vi "Untitled 1.vi"() -> ()   [LabVIEW 2017]
uses:
  <vilib>/xml/Load XML String.vi
  <vilib>/xml/Close Reference(Node).vi
  <vilib>/addons/internet/NI_InternetTK_Core_VIs.lvlib
  <vilib>/xml/NI_XML.lvlib
  <resource>/objmgr/DOMUserDefRef.rc
panel:
  out "I, J,K,X, Y,Z":dbl[](array[numeric])
  out "content":string
  out "concatenated string":string
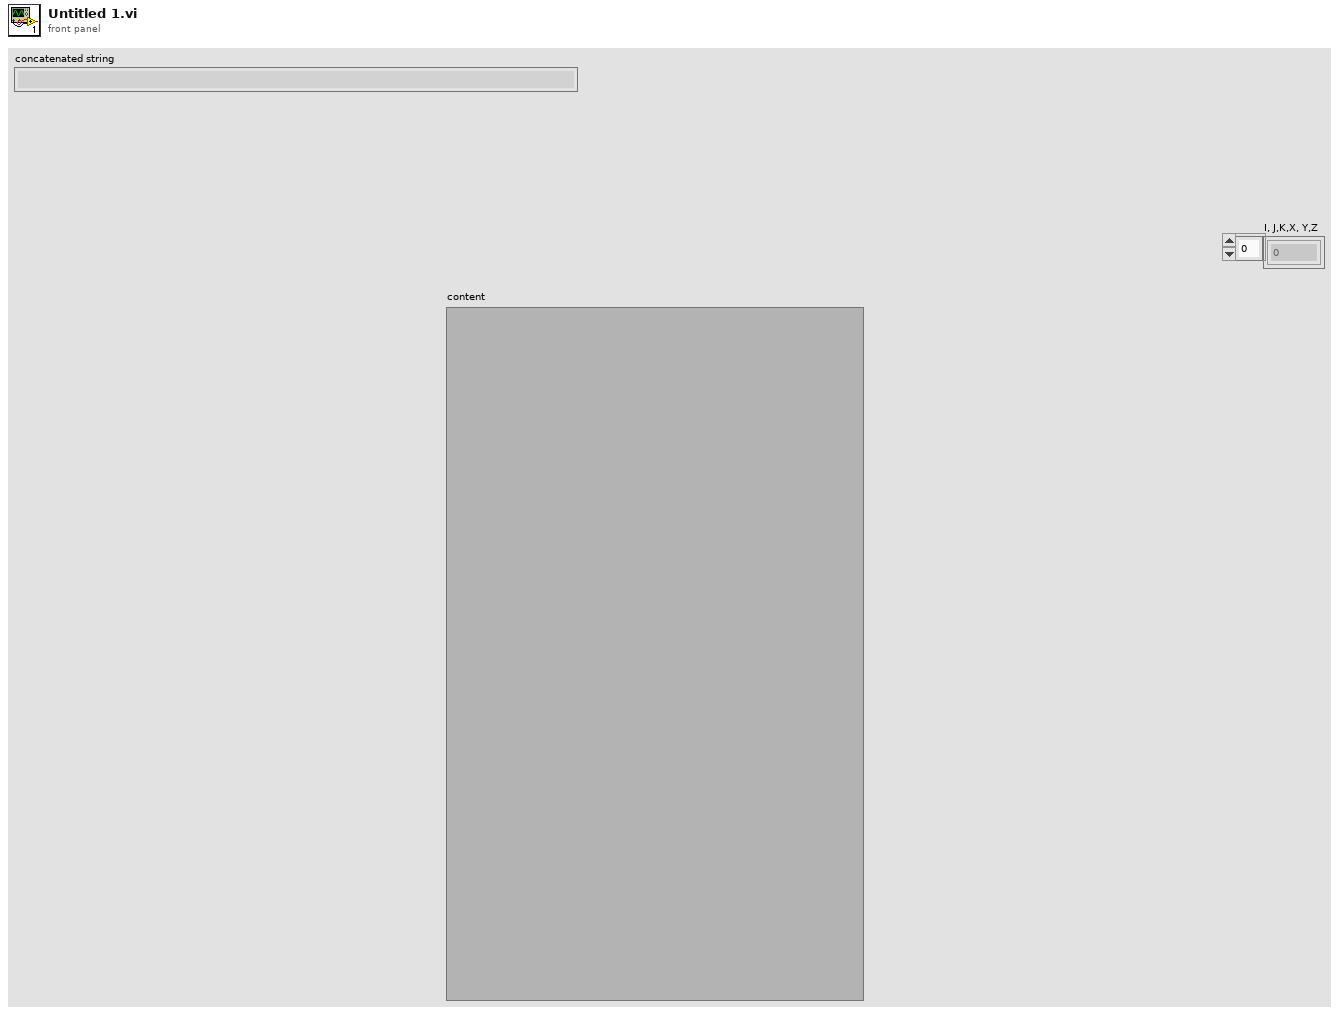
[diagram p1: front panel]
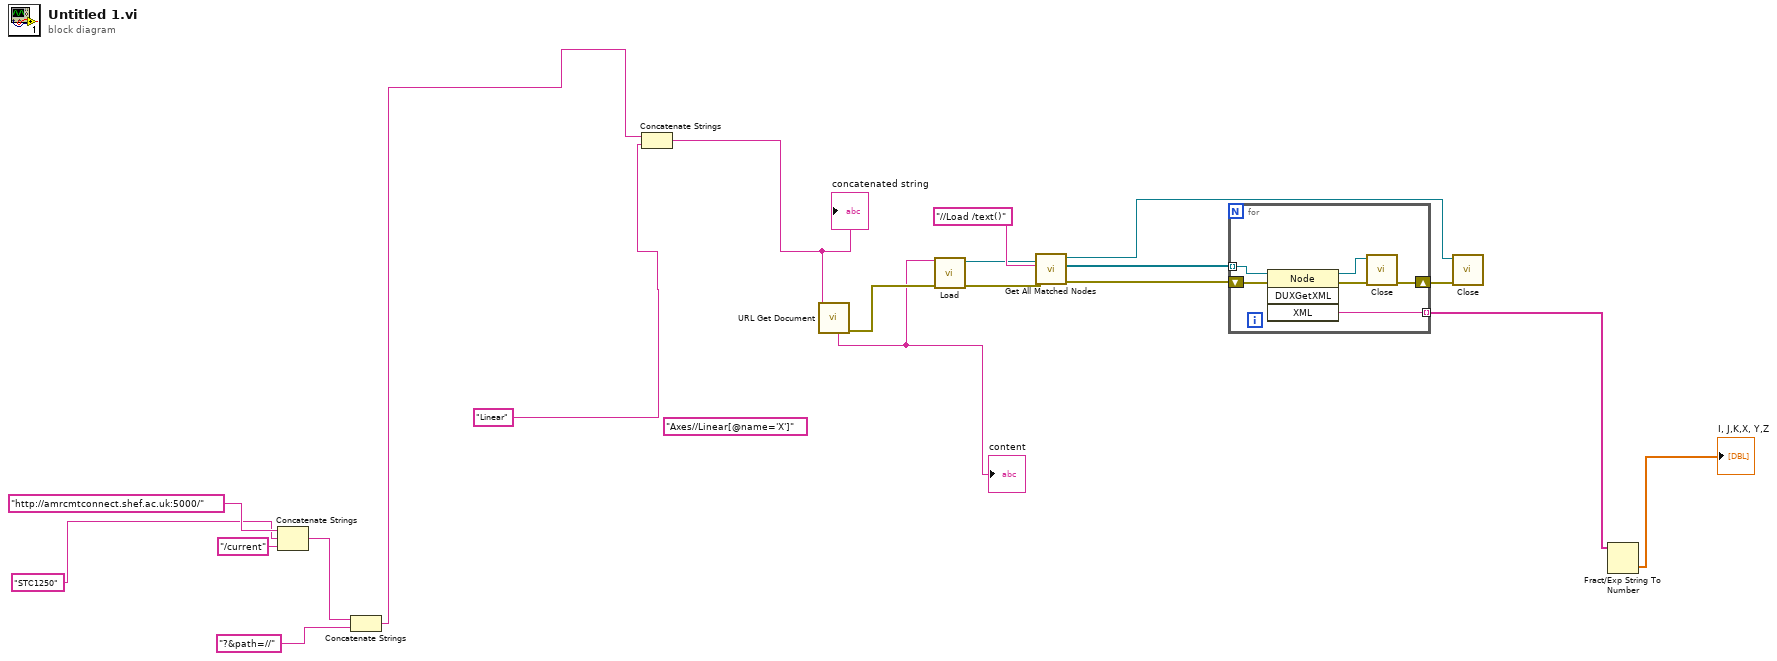
[diagram p0: block diagram]
diagram:
  (unwired) "Axes//Linear[@name='X']" ("URL")
  n1 = Concatenate Strings("http://amrcmtconnect.shef.ac.uk:5000/" ("MT Connect Agent"), "STC1250" ("Machine"), "/current" ("string")) -> (w3:string)
  n2 = Concatenate Strings(w3, "?&path=//" ("string")) -> (w1:string)
  n3 = Concatenate Strings(w1, "Linear" ("URL")) -> (w11:string)
  "concatenated string" <- w11
  n4 = call <vilib>:"URL Get Document.vi"("URL"=w11) -> ("error out"=w19:errorcluster, "content"=w10:string)  [unwired: 6 in, 3 out]
  "content" <- w10
  n5 = call-poly <vilib>:"Load.vi"("XML string"=w10, "error in (no error)"=w19) -> ("DOM document out"=w15:refnum<k20>, "error out"=w16:errorcluster)  [unwired: 11 in, 1 out]
  n6 = call <vilib>:"Get All Matched Nodes.vi"("error in (no error)"=w16, "XPath expression"="//Load /text()", "node in"=w15) -> ("error out"=w13:errorcluster, "node result array"=w12:refnum<k20>[], "node out"=w17:refnum<k20>)  [unwired: 6 out]
  n7 = for {
    tunnel: w12 -> [w21] mode=indexing
    shift-right: [w23] -> w14
    shift-left: w13 -> [w22]
    tunnel: [w20] -> w8 mode=indexing
    n8 = invoke on="Invoke Node" class="Node" method="DUXGetXML"(reference=w21, error in=w22) -> (reference out=w24:refnum<k20>, error out=w25:errorcluster, "XML"=w20:string)  [unwired: 2 in, 1 out]
    n9 = call-poly <vilib>:"Close.vi"("error in (no error)"=w25, "node"=w24) -> ("error out"=w23:errorcluster)  [unwired: 7 out]
  }
  n10 = call-poly <vilib>:"Close.vi"("error in (no error)"=w14, "node"=w17) -> ()  [unwired: 8 out]
  n11 = Fract/Exp String To Number(string=w8) -> (number=→"I, J,K,X, Y,Z":dbl[])  [unwired: 3 in, 1 out]
